vi "Adjust ADCs Persona.vi"(5 "CustomCal?":bool, 7 "Original CalData":dbl[][](array[numeric]), 8 "Recal?":bool, 9 "Clear?":bool, 11 "Live Raw USB data":u16[](array[numeric])) -> (3 "LiveData":T1 {"Reference/Temperature 2" format="%.2f"; "Accelerometer" format="%.2f"; "Battery" format="%.2f"; "Reference/Temperature 1" format="%.2f"; "LoadSensors" format="%.2f"})   [LabVIEW 2015]
uses:
  Controls/LiveData.ctl
  Controls/SignalProcess.ctl
  Controls/Gen2 FT Globals.vi
panel:
  out "transposed array":dbl[][](array[numeric])
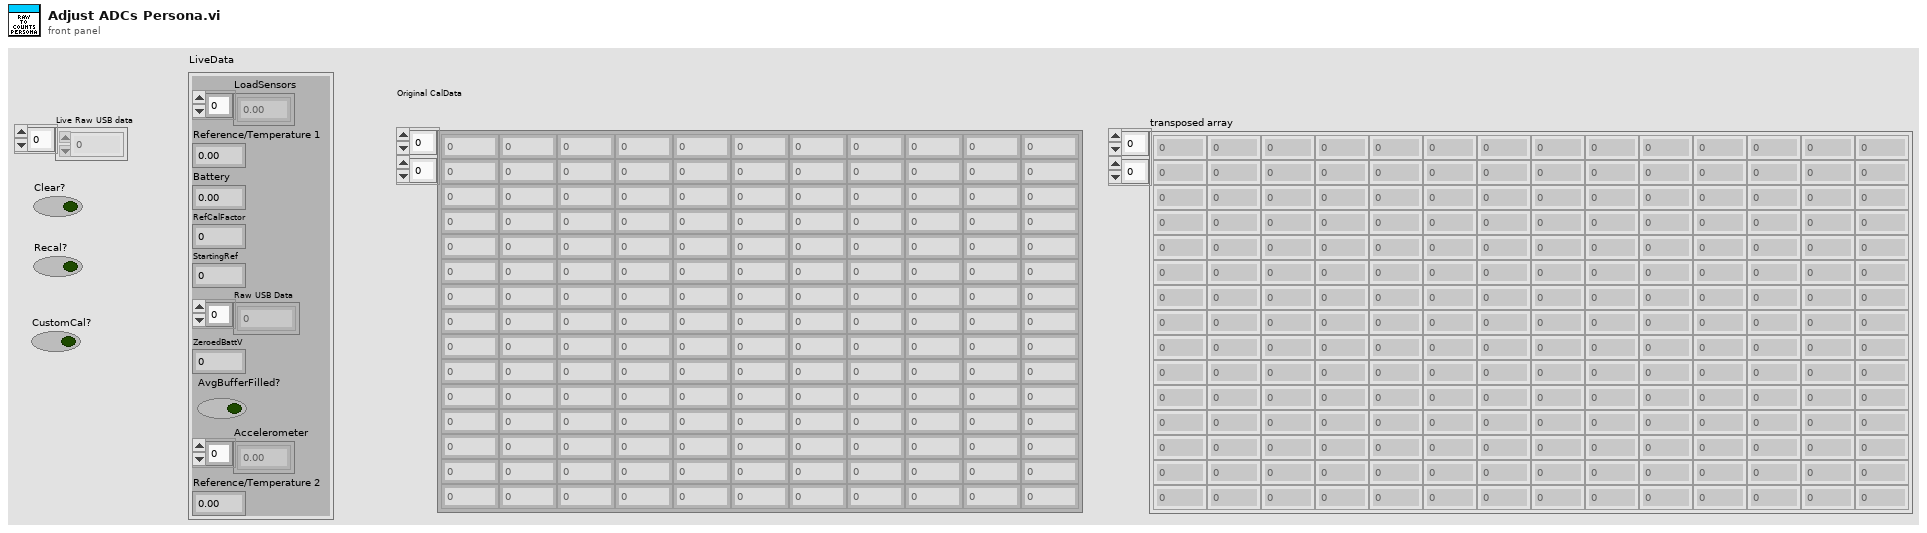
[diagram p1: front panel]
types:
  T1 = typedef "LiveData.ctl" = cluster{"LoadSensors":dbl[], "Reference/Temperature 1":dbl, "Battery":dbl, "RefCalFactor":dbl, "StartingRef":dbl, "Raw USB Data":u16[], "ZeroedBattV":dbl, "AvgBufferFilled?":bool, "Accelerometer":dbl[], "Reference/Temperature 2":dbl}
  T2 = typedef "SignalProcess.ctl" = enum16{"Remove Duplicates", "Adjust Channels", "Filter Signal", "Fill Average Array", "Recalibrate", "Calibrate Accelerometers", "Adjust Against Ref", "Timeout"}
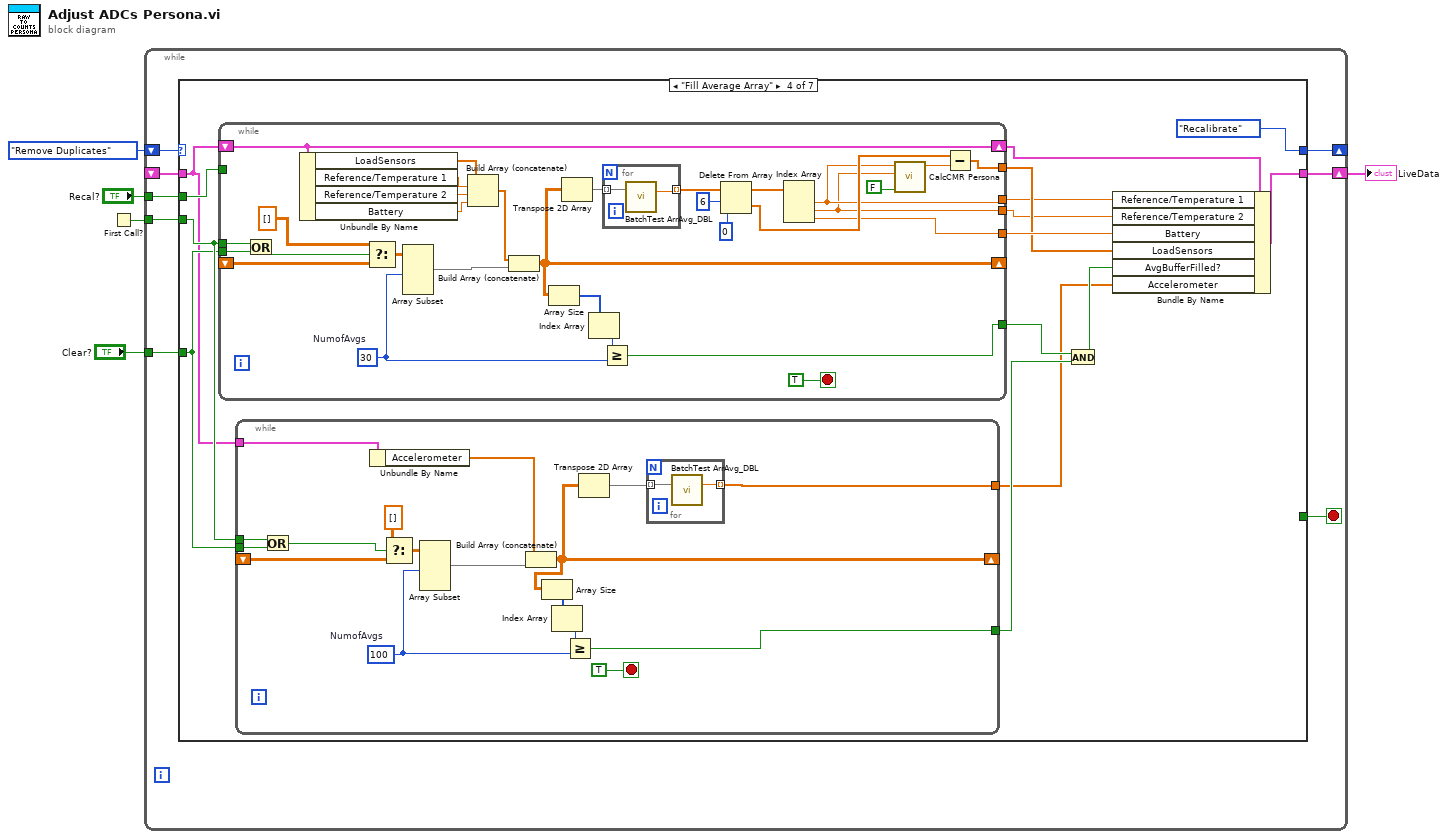
[diagram p0: block diagram]
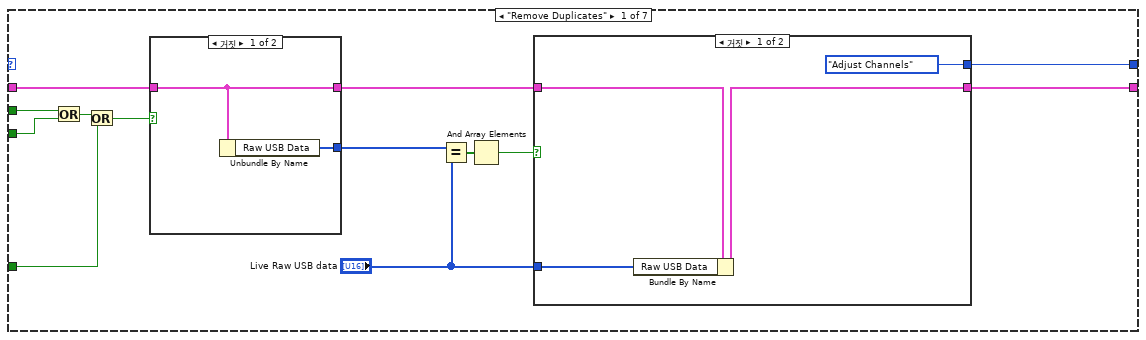
[diagram p2: hidden frame]
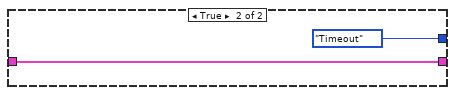
[diagram p3: hidden frame]
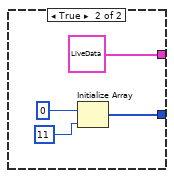
[diagram p4: hidden frame]
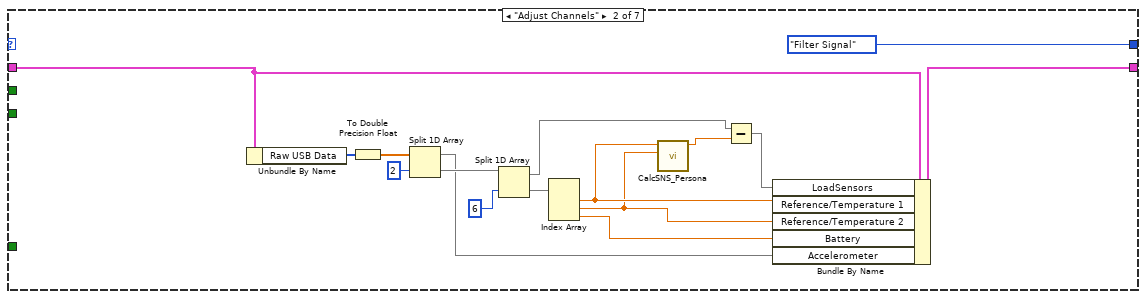
[diagram p5: hidden frame]
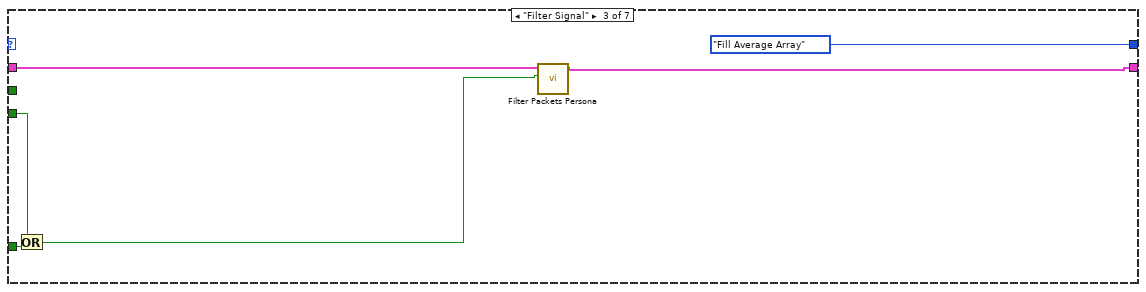
[diagram p6: hidden frame]
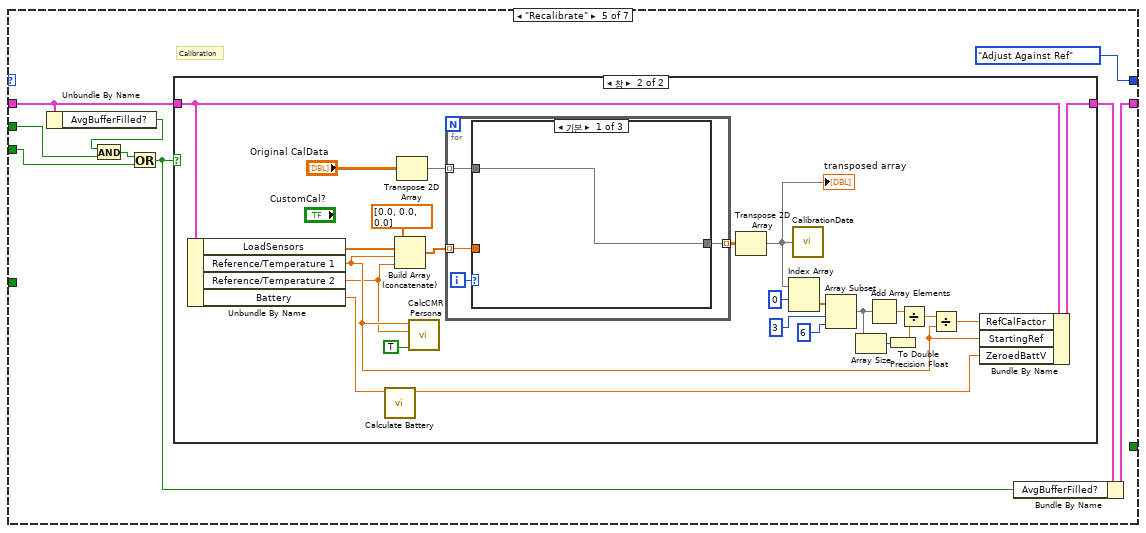
[diagram p7: hidden frame]
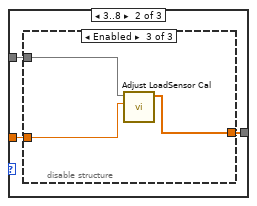
[diagram p9: hidden frame]
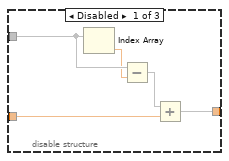
[diagram p10: hidden frame]
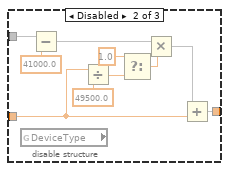
[diagram p11: hidden frame]
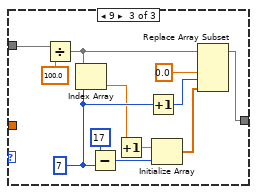
[diagram p12: hidden frame]
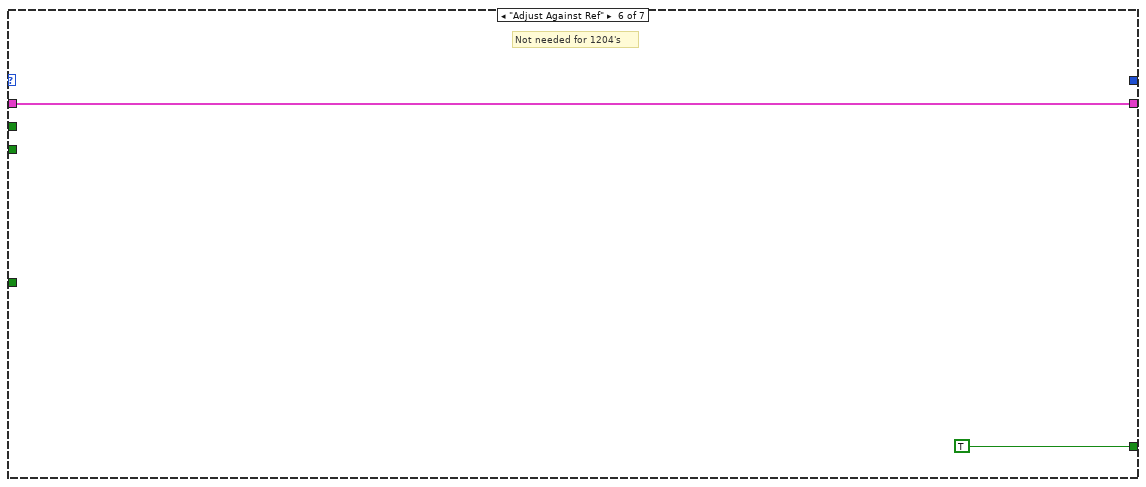
[diagram p13: hidden frame]
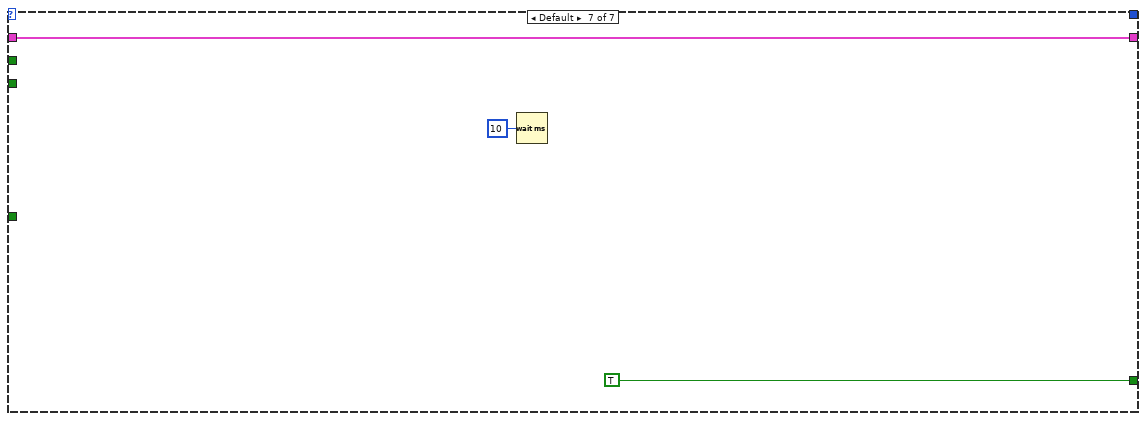
[diagram p14: hidden frame]
diagram:
  n1 = First Call?() -> (First Call?: T/F=w4:bool)
  n2 = while {
    shift-right: [w13] -> w2
    shift-left: _ -> [w10]
    shift-right: [w11] -> _
    shift-left: SignalProcess."Remove Duplicates" -> [w12]
    tunnel: w4 -> [w8]
    tunnel: "Recal?" -> [w7]
    tunnel: "Clear?" -> [w6]
    stop <- w9 stop-if-true
    n3 = case shown="\"Fill Average Array\"" w12 {
      tunnel: [w19 w48 w55 w64 w129 w200 w204] -> w13
      tunnel: [w21 SignalProcess."Filter Signal" SignalProcess."Fill Average Array" SignalProcess."Recalibrate" ("f") SignalProcess."Adjust Against Ref" _ _] -> w11
      tunnel: w10 -> [w26 w49 w57 w71 w131 w200 w204]
      tunnel: [_ _ _ _ _ TRUE TRUE] -> w9
      tunnel: w8 -> [w18 _ w59 w73 w135 _ _]
      tunnel: w7 -> [w25 _ _ w74 w136 _ _]
      tunnel: w6 -> [w14 _ w58 w72 _ _ _]
      frame "Remove Duplicates" {
        n4 = Or(x=w25, y=w18) -> (x .or. y?=w15:bool)
        n5 = Or(x=w15, y=w14) -> (x .or. y?=w16:bool)
        n6 = case shown="거짓" w16 {
          tunnel: [w34 T1 {"LoadSensors"=[], "Reference/Temperature 1"=0.0, "Battery"=0.0, "RefCalFactor"=0.0, "StartingRef"=0.0, "Raw USB Data"=[], "ZeroedBattV"=0.0, "AvgBufferFilled?"=FALSE, "Accelerometer"=[], "Reference/Temperature 2"=0.0} ("LiveData")] -> w20
          tunnel: w26 -> [w34 _]
          tunnel: [w33 w36] -> w24
          frame False {
            n7 = Unbundle By Name(w34) -> ("Raw USB Data"=w33:u16[])
          }
          frame True {
            n8 = Initialize Array(u16 0 ("element"), 11 ("dimension size")) -> (w36:u16[])
          }
        }
        n9 = Equal?(x=w24, y="Live Raw USB data") -> (x = y?=w23:bool[])
        n10 = And Array Elements(Boolean array=w23) -> (logical AND=w22:bool)
        n11 = case shown="거짓" w22 {
          tunnel: [SignalProcess."Adjust Channels" SignalProcess."Timeout"] -> w21
          tunnel: "Live Raw USB data" -> [w27 _]
          tunnel: w20 -> [w29 w31]
          tunnel: [w28 w31] -> w19
          frame False {
            n12 = Bundle By Name(cluster=w29, "Raw USB Data"=w27) -> (w28:T1)
          }
          frame True {
          }
        }
      }
      frame "Adjust Channels" {
        n13 = Unbundle By Name(w49) -> ("Raw USB Data"=w47:u16[])
        n14 = To Double Precision Float(number=w47) -> (double precision float=w46:dbl[])
        n15 = Split 1D Array(array=w46, index=2) -> (first subarray=w43:dbl[], second subarray=w53:dbl[])
        n16 = Split 1D Array(array=w53, index=6) -> (first subarray=w45:dbl[], second subarray=w51:dbl[])
        n17 = Index Array(array=w51) -> (element #1=w41:dbl, element #2=w40:dbl, element #3=w42:dbl)  [unwired: 3 in]
        n18 = call "CalcSNS_Persona.vi"("Ref Sensor 2"=w40, "Ref Sensor"=w41) -> ("delta SNS"=w39:dbl)  [unwired: 9 in]
        n19 = Subtract(x=w45, y=w39) -> (x-y=w44:dbl[])
        n20 = Bundle By Name(cluster=w49, "LoadSensors"=w44, "Reference/Temperature 1"=w41, "Reference/Temperature 2"=w40, "Battery"=w42, "Accelerometer"=w43) -> (w48:T1)
      }
      frame "Filter Signal" {
        n21 = Or(x=w59, y=w58) -> (x .or. y?=w56:bool)
        n22 = call "Filter Packets Persona.vi"("Boolean"=w56, "LiveData in"=w57) -> ("LiveData out"=w55:T1)  [unwired: 9 in]
      }
      frame "Fill Average Array" {
        n23 = while {
          shift-right: [w105] -> _
          shift-left: _ -> [w111]
          shift-right: [w101] -> w63
          shift-left: w71 -> [w101]
          tunnel: w73 -> [w115]
          tunnel: w74 -> [_]
          tunnel: w72 -> [w114]
          tunnel: [w98] -> w62
          tunnel: [w99] -> w70
          tunnel: [w103] -> w69
          tunnel: [w102] -> w66
          tunnel: [w96] -> w61
          stop <- TRUE stop-if-true
          w109 = 30  # NumofAvgs
          n24 = Or(x=w115, y=w114) -> (x .or. y?=w112:bool)
          n25 = Unbundle By Name(w101) -> ("LoadSensors"=w124:dbl[], "Reference/Temperature 1"=w123:dbl, "Reference/Temperature 2"=w122:dbl, "Battery"=w100:dbl)
          n26 = Select(t=dbl[][] [], s=w112, f=w111) -> (s? t:f=w110:dbl[][])
          n27 = Array Subset(array=w110, length (row)=w109) -> (w108:dbl[][])  [unwired: 3 in]
          n28 = Build Array (concatenate)(w124, w123, w122, w100) -> (w107:dbl[])
          n29 = Build Array (concatenate)(w107, w108) -> (w105:dbl[][])
          n30 = Array Size(array=w105) -> (size(s)=w118:i32[])
          n31 = Transpose 2D Array(2D array=w105) -> (transposed array=w106:dbl[][])
          n32 = Index Array(array=w118) -> (element=w117:i32)  [unwired: 1 in]
          n33 = Greater Or Equal?(x=w117, y=w109) -> (x >= y?=w102:bool)
          n34 = for {
            tunnel: w106 -> [w127] mode=indexing
            tunnel: [w126] -> w116 mode=indexing
            n35 = call "BatchTest ArrAvg_DBL.vi"("Array In"=w127) -> ("Average"=w126:dbl)  [unwired: 14 in]
          }
          n36 = Delete From Array(array=w116, length=6, index=0) -> (deleted portion=w104:dbl[], array with subset deleted=w119:dbl[])
          n37 = Index Array(array=w119) -> (element #1=w98:dbl, element #2=w96:dbl, element #3=w99:dbl)  [unwired: 3 in]
          n38 = call "CalcCMR Persona.vi"("Zero?"=FALSE, "Ref Sensor 2"=w96, "Ref Sensor"=w98) -> ("delta SNS"=w95:dbl)  [unwired: 8 in]
          n39 = Subtract(x=w104, y=w95) -> (x-y=w103:dbl[])
        }
        n40 = while {
          shift-right: [w81] -> _
          shift-left: _ -> [w85]
          tunnel: w73 -> [w89]
          tunnel: w72 -> [w88]
          tunnel: w71 -> [w79]
          tunnel: [w78] -> w68
          tunnel: [w77] -> w65
          stop <- TRUE stop-if-true
          w83 = 100  # NumofAvgs
          n41 = Or(x=w89, y=w88) -> (x .or. y?=w86:bool)
          n42 = Unbundle By Name(w79) -> ("Accelerometer"=w80:dbl[])
          n43 = Select(t=dbl[][] [], s=w86, f=w85) -> (s? t:f=w84:dbl[][])
          n44 = Array Subset(array=w84, length (row)=w83) -> (w82:dbl[][])  [unwired: 3 in]
          n45 = Build Array (concatenate)(w80, w82) -> (w81:dbl[][])
          n46 = Array Size(array=w81) -> (size(s)=w91:i32[])
          n47 = Index Array(array=w91) -> (element=w90:i32)  [unwired: 1 in]
          n48 = Greater Or Equal?(x=w90, y=w83) -> (x >= y?=w78:bool)
          n49 = Transpose 2D Array(2D array=w81) -> (transposed array=w76:dbl[][])
          n50 = for {
            tunnel: w76 -> [w94] mode=indexing
            tunnel: [w93] -> w77 mode=indexing
            n51 = call "BatchTest ArrAvg_DBL.vi"("Array In"=w94) -> ("Average"=w93:dbl)  [unwired: 14 in]
          }
        }
        n52 = And(x=w66, y=w68) -> (x .and. y?=w67:bool)
        n53 = Bundle By Name(cluster=w63, "Reference/Temperature 1"=w62, "Reference/Temperature 2"=w61, "Battery"=w70, "LoadSensors"=w69, "AvgBufferFilled?"=w67, "Accelerometer"=w65) -> (w64:T1)
      }
      frame "Recalibrate" {
        # "Calibration"
        n54 = Unbundle By Name(w131) -> ("AvgBufferFilled?"=w130:bool)
        n55 = And(x=w130, y=w136) -> (x .and. y?=w132:bool)
        n56 = Or(x=w132, y=w135) -> (x .or. y?=w128:bool)
        n57 = case shown="참" w128 {
          tunnel: w131 -> [w137 w152]
          tunnel: [w137 w148] -> w133
          frame False {
          }
          frame True {
            n58 = Unbundle By Name(w152) -> ("LoadSensors"=w142:dbl[], "Reference/Temperature 1"=w140:dbl, "Reference/Temperature 2"=w139:dbl, "Battery"=w141:dbl)
            n59 = call "Calculate Battery.vi"("Battery A/D in"=w141) -> ("Battery Volts Out"=w147:dbl)  [unwired: 10 in]
            n60 = Build Array (concatenate)(dbl[] [0.0, 0.0, 0.0], w142, w140, w139) -> (w145:dbl[])
            n61 = Transpose 2D Array(2D array="Original CalData") -> (transposed array=w146:dbl[][])
            n62 = call "CalcCMR Persona.vi"("Zero?"=TRUE, "Ref Sensor 2"=w139, "Ref Sensor"=w140) -> ()  [unwired: 8 in, 1 out]
            n63 = for {
              tunnel: w146 -> [w165] mode=indexing
              tunnel: w145 -> [w162] mode=indexing
              tunnel: [w164] -> w143 mode=indexing
              i -> [w163]
              n64 = case shown="기본" w163 {
                tunnel: w162 -> [_ w168 _]
                tunnel: w165 -> [w166 w169 w193]
                tunnel: [w166 w167 w195] -> w164
                frame Default {
                }
                frame 3..8 {
                  n65 = disable-structure shown="Enabled" {
                    disable-tunnel: w169 -> [w174 w184 w187]
                    disable-tunnel: w168 -> [w171 w175 w185]
                    disable-tunnel: [w170 w182 w186] -> w167
                    frame Disabled {
                      n66 = Index Array(array=w174) -> (element=w173:dbl)  [unwired: 1 in]
                      n67 = Subtract(x=w174, y=w173) -> (x-y=w172:dbl[])
                      n68 = Add(x=w172, y=w171) -> (x+y=w170:dbl[])
                    }
                    frame Disabled {
                      n69 = global read "Gen2 FT Globals.vi" "DeviceType"() -> ()  [unwired: 1 out]
                      n70 = Subtract(x=w184, y=41000.0 ("element")) -> (x-y=w183:dbl[])
                      n71 = Divide(x=w175, y=49500.0) -> (x/y=w177:dbl)
                      n72 = Select(t=1.0, f=w177) -> (s? t:f=w176:dbl)  [unwired: 1 in]
                      n73 = Multiply(x=w183, y=w176) -> (x*y=w180:dbl[])
                      n74 = Add(x=w180, y=w175) -> (x+y=w182:dbl[])
                    }
                    frame Enabled {
                      n75 = call "Adjust LoadSensor Cal.vi"("0_Load"=w185, "LS CalData In"=w187) -> ("LS CalData Out"=w186:dbl[])  [unwired: 9 in]
                    }
                  }
                }
                frame 9 {
                  w191 = 7 ("index of element")
                  n76 = Divide(x=w193, y=100.0) -> (x/y=w188:dbl[])
                  n77 = Index Array(array=w188, index=w191) -> (element=w189:dbl)
                  n78 = Subtract(x=17 ("dimension size"), y=w191) -> (x-y=w198:i32)
                  n79 = Increment(x=w189) -> (x+1=w199:dbl)
                  n80 = Increment(x=w191) -> (x+1=w190:i32)
                  n81 = Initialize Array(w199, w198) -> (w192:dbl[])
                  n82 = Replace Array Subset(array=w188, new element #1=0.0 ("new element/subarray"), new element #2=w192, index #2=w190) -> (w195:dbl[])  [unwired: 1 in]
                }
              }
            }
            n83 = Transpose 2D Array(2D array=w143) -> (transposed array=w151:dbl[][])
            "transposed array" <- w151
            n84 = Index Array(array=w151, index (row)=0) -> (element=w154:dbl[])  [unwired: 1 in]
            n85 = call "CalibrationData.vi"("CalData In"=w151) -> ()  [unwired: 1 out]
            n86 = Array Subset(array=w154, index=3, length=6) -> (w155:dbl[])
            n87 = Array Size(array=w155) -> (size(s)=w157:i32)
            n88 = Add Array Elements(numeric array=w155) -> (sum=w158:dbl)
            n89 = To Double Precision Float(number=w157) -> (double precision float=w156:dbl)
            n90 = Divide(x=w158, y=w156) -> (x/y=w153:dbl)
            n91 = Divide(x=w153, y=w140) -> (x/y=w149:dbl)
            n92 = Bundle By Name(cluster=w152, "RefCalFactor"=w149, "StartingRef"=w140, "ZeroedBattV"=w147) -> (w148:T1)
          }
        }
        n93 = Bundle By Name(cluster=w133, "AvgBufferFilled?"=w128) -> (w129:T1)
      }
      frame "Adjust Against Ref" {
        # "Not needed for 1204's"
      }
      frame Default {
        n94 = Wait (ms)(milliseconds to wait=u32 10) -> ()  [unwired: 1 out]
      }
    }
  }
  "LiveData" <- w2
